vi "MakeSortable.vi"(1 "string in":string) -> (0 "string out":string)   [LabVIEW 2024]
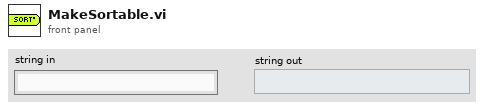
[diagram p1: front panel]
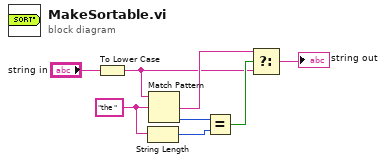
[diagram p0: block diagram]
diagram:
  w2 = "the " ("regular expression")
  n1 = To Lower Case(string="string in") -> (all lower case string=w4:string)
  n2 = String Length(string=w2) -> (length=w1:i32)
  n3 = Match Pattern(string=w4, regular expression=w2) -> (after substring=w5:string, offset past match=w7:i32)  [unwired: 1 in, 2 out]
  n4 = Equal?(x=w7, y=w1) -> (x = y?=w6:bool)
  n5 = Select(t=w5, s=w6, f=w4) -> (s? t:f=→"string out":string)
